vi "Select NIM.vi"() -> ()   [LabVIEW 2024]
uses:
  <vilib>/addons/database/Connection.llb/Conn ObjectReference.ctl
  <vilib>/addons/database/Connection.llb/Conn Execute.vi
  <vilib>/addons/database/NI_Database_API.lvlib
panel:
  in  "Boolean":bool
  out "error out":errorcluster
  out "connection reference 2":T1
  in  "error in (no error)":errorcluster
  in  "connection reference":T1
  in  "string":string
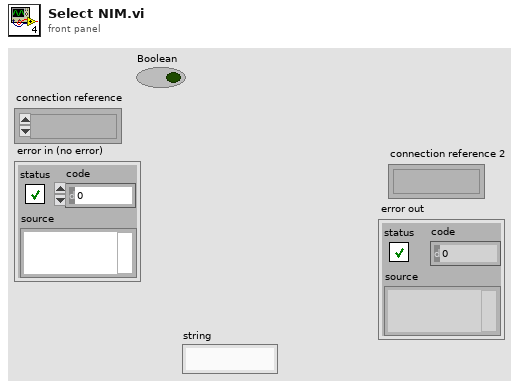
[diagram p1: front panel]
types:
  T1 = typedef "NI_Database_API.lvlib/Conn ObjectReference.ctl" = refnum<k1>
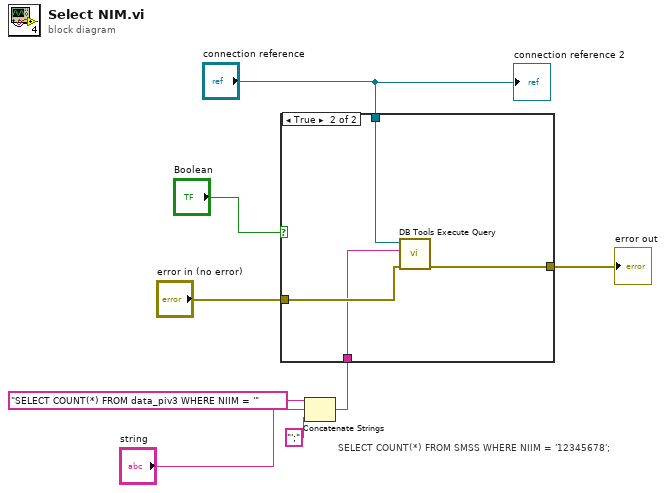
[diagram p0: block diagram]
diagram:
  # "SELECT COUNT(*) FROM SMSS WHERE NIIM = '12345678';"
  n1 = Concatenate Strings("SELECT COUNT(*) FROM data_piv3 WHERE NIIM = '", "string", "';" ("string")) -> (w1:string)
  n2 = case shown="True" "Boolean" {
    tunnel: "connection reference" -> [_ w13]
    tunnel: "error in (no error)" -> [w9 w12]
    tunnel: [w9 w11] -> w3
    tunnel: w1 -> [_ w10]
    frame False {
    }
    frame True {
      n3 = call-poly <vilib>:"DB Tools Execute Query.vi"("error in (no error)"=w12, "SQL query"=w10, "connection reference"=w13) -> ("error out"=w11:errorcluster)  [unwired: 5 in, 1 out]
    }
  }
  "error out" <- w3
  "connection reference 2" <- "connection reference"
